vi "LUnit Configure.vi"(8 "error in (no error)":errorcluster, 9 "Default Path":path, 10 "Interactive?":bool, 11 "Coverage Report In":refnum<class "Coverage Report.lvclass">) -> (0 "error out":errorcluster, 3 "Coverage Report Out":refnum<class "Coverage Report.lvclass">)   [LabVIEW 2020, in "Coverage Report.lvclass"]
uses:
  Coverage Report.lvclass
  Coverage Report.lvclass/Coverage Report.ctl
  f97740a0-8655-44de-873d-fc598e584b33.vi
  <vilib>/Astemes/LUnit/Framework/LUnit Configuration Manager.lvclass
  <vilib>/Astemes/DevEnv/Styling/Color Theme.lvlib
panel:
  in  "VI tree":string[](tree)
  out "Coverage Include File Path":path
  in  "Report Path":path
  in  "Cancel":bool
  in  "Open New Reports":bool
  in  "Open Result in UI":bool
  in  "Commit":bool
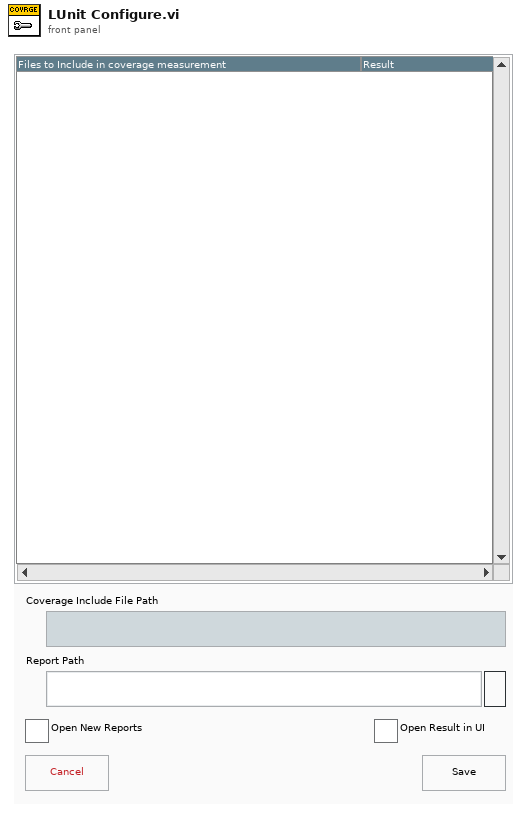
[diagram p1: front panel]
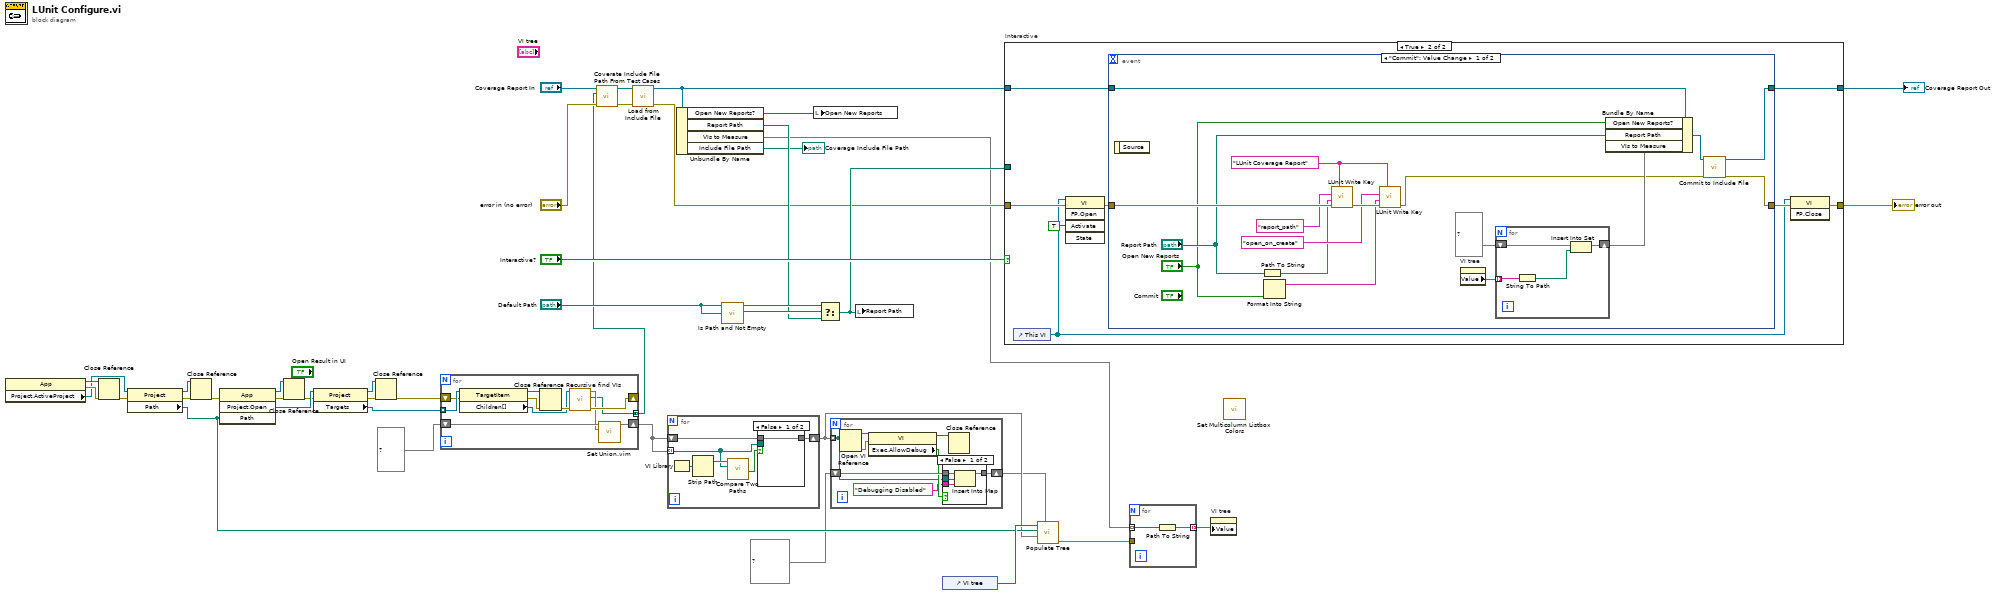
[diagram p0: block diagram]
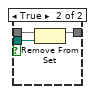
[diagram p3: hidden frame]
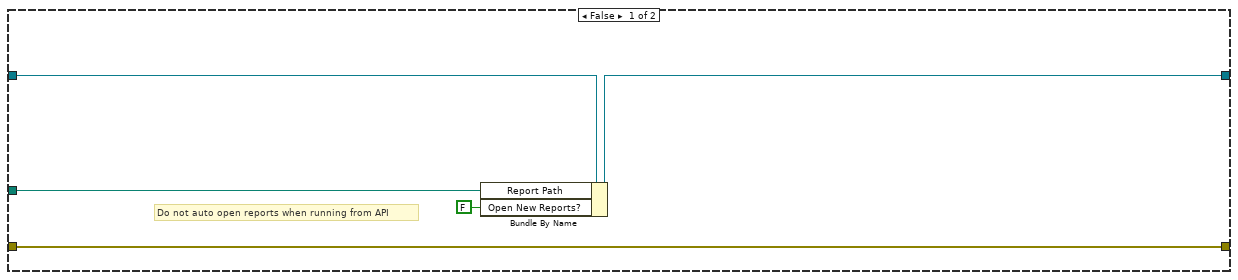
[diagram p4: hidden frame]
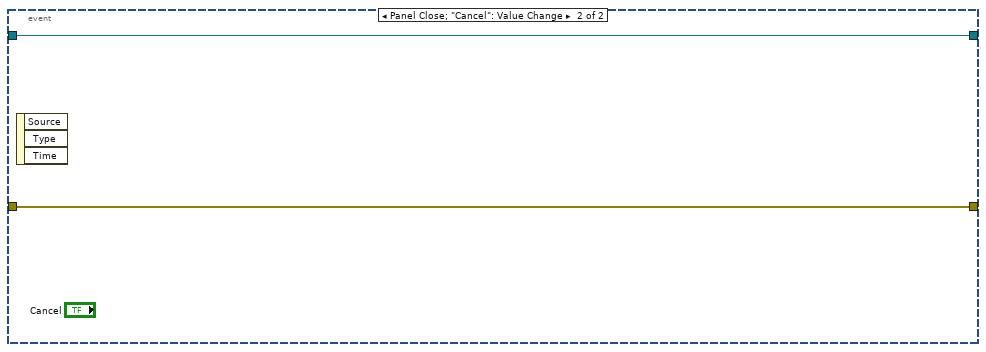
[diagram p5: hidden frame]
diagram:
  n1 = property class="App"() -> (reference out=w19:refnum<vi>, error out=w22:errorcluster, "Project.ActiveProject"=w18:refnum<vi>)  [unwired: 2 in]
  n2 = Close Reference(reference=w19, error in (no error)=w22) -> (error out=w23:errorcluster)
  n3 = property class="Project"(reference=w18, error in=w23) -> (reference out=w20:refnum<vi>, error out=w21:errorcluster, "Path"=w5:path)
  n4 = Close Reference(reference=w20, error in (no error)=w21) -> (error out=w24:errorcluster)
  n5 = invoke class="App" method="Project.Open"(error in=w24, "Path"=w5) -> (reference out=w27:refnum<vi>, error out=w31:errorcluster, "Project:Open"=w33:refnum<vi>)  [unwired: 2 in, 1 out]
  n6 = Close Reference(reference=w27, error in (no error)=w31) -> (error out=w28:errorcluster)
  n7 = property class="Project"(reference=w33, error in=w28) -> (reference out=w29:refnum<vi>, error out=w32:errorcluster, "Targets"=w25:refnum<vi>[])
  n8 = Close Reference(reference=w29, error in (no error)=w32) -> (error out=w30:errorcluster)
  n9 = for {
    tunnel: w25 -> [w52] mode=indexing
    shift-right: [w49] -> _
    shift-left: w30 -> [w50]
    shift-right: [w45] -> w8
    shift-left: set{path} {} ("VIs") -> [w47]
    tunnel: [w42] -> w11 mode=concatenating
    n10 = property class="TargetItem"(reference=w52, error in=w50) -> (reference out=w48:refnum<vi>, error out=w51:errorcluster, "Children[]"=w43:refnum<vi>[])
    n11 = Close Reference(reference=w48, error in (no error)=w51) -> (error out=w44:errorcluster)
    n12 = call "Recursive find VIs.vi"("error in (no error)"=w44, "Project Items"=w43) -> ("error out"=w49:errorcluster, "Test Case Classes"=w42:path[], "VIs"=w46:set{path})  [unwired: 7 in]
    n13 = call "Set Union.vim"("set 2"=w46, "set 1"=w47) -> ("union"=w45:set{path})  [unwired: 9 in]
  }
  n14 = call "Coverate Include File Path From Test Cases.vi"("error in (no error)"="error in (no error)", "Test Case Classes"=w11, "Coverage Report.lvclass"="Coverage Report In") -> ("error out"=w16:errorcluster, "Coverage Report.lvclass 2"=w17:refnum<class "Coverage Report.lvclass">)  [unwired: 7 in]
  n15 = call "Load from Include File.vi"("error in (no error)"=w16, "Coverage Report in"=w17) -> ("error out"=w12:errorcluster, "Coverage Report out"=w14:refnum<class "Coverage Report.lvclass">)  [unwired: 8 in]
  n16 = for {
    tunnel: w8 -> [w55] mode=indexing
    shift-right: [w54] -> w3
    shift-left: w8 -> [w56]
    n17 = VI Library() -> (path=w57:path)
    n18 = Strip Path(path=w57) -> (stripped path=w58:path)  [unwired: 1 out]
    n19 = call <vilib>:"Compare Two Paths.vi"("Path 2"=w55, "Path 1"=w58) -> ("Path 2 Relative to Path 1?"=w53:bool)  [unwired: 6 in, 3 out]
    n20 = case shown="False" w53 {
      tunnel: w56 -> [w59 w62]
      tunnel: w55 -> [_ w61]
      tunnel: [w59 w60] -> w54
      frame False {
      }
      frame True {
        n21 = Remove From Set(10:w61, 11:w62) -> (3:w60:set{path})  [unwired: 1 out]
      }
    }
  }
  n22 = Unbundle By Name(w14) -> ("Open New Reports?"=w34:bool, "Report Path"=w35:path, "VIs to Measure"=w6:set{path}, "Include File Path"=→"Coverage Include File Path":path)
  n23 = call <vilib>:"Is Path and Not Empty.vi"("path"="Default Path") -> ("Is Path and Not Empty?"=w38:bool)  [unwired: 4 in]
  n24 = local write "Open New Reports"(w34) -> ()
  n25 = Select(t="Default Path", s=w38, f=w35) -> (s? t:f=w37:path)
  n26 = for {
    tunnel: w3 -> [w64] mode=indexing
    shift-right: [w65] -> w1
    shift-left: map{path, string} {} ("Results") -> [w69]
    n27 = Open VI Reference(vi path=w64) -> (vi reference=w70:refnum<vi>, error out=w67:errorcluster)  [unwired: 5 in]
    n28 = property class="VI"(reference=w70, error in=w67) -> (reference out=w68:refnum<vi>, "Exec.AllowDebug"=w66:bool)  [unwired: 1 out]
    n29 = case shown="False" w66 {
      tunnel: w69 -> [w74 w75]
      tunnel: [w73 w75] -> w65
      tunnel: w64 -> [w72 _]
      tunnel: "Debugging Disabled" ("value") -> [w71 _]
      frame False {
        n30 = Insert Into Map(map in=w74, key=w72, value=w71) -> (map out=w73:map{path, string})  [unwired: 2 out]
      }
      frame True {
      }
    }
    n31 = Close Reference(reference=w68) -> ()  [unwired: 1 in, 1 out]
  }
  n32 = local write "Report Path"(w37) -> ()
  n33 = control-ref of="VI tree"() -> (w9:refnum<vi>)
  n34 = case "Interactive" shown="True" "Interactive?" {
    tunnel: w12 -> [w80 w86]
    tunnel: [w80 w84] -> w41
    tunnel: w14 -> [w79 w81]
    tunnel: [w78 w82] -> w39
    tunnel: w37 -> [w77 _]
    frame False {
      # "Do not auto open reports when running from API"
      n35 = Bundle By Name(cluster=w79, "Report Path"=w77, "Open New Reports?"=FALSE) -> (w78:refnum<class "Coverage Report.lvclass">)
    }
    frame True {
      n36 = control-ref of="This VI"() -> (w83:refnum<vi>)
      n37 = invoke class="VI" method="FP.Open"(reference=w83, error in=w86, "Activate"=TRUE ("Activate?")) -> (error out=w87:errorcluster)  [unwired: 2 in, 4 out]
      n38 = event shown="[0] \"Commit\": Value Change" {
        selector: _ -> [_ _]
        dyn-events: _ -> [_ _]
        timeout: _ -> [_ _]
        tunnel: w87 -> [w105 w111]
        tunnel: [w92 w111] -> w85
        tunnel: w81 -> [w99 w110]
        tunnel: [w93 w110] -> w82
        event "Commit": Value Change {
          w90 = "LUnit Coverage Report"
          n39 = event-data() -> ()  [unwired: 1 in, 1 out]
          n40 = Path To String(path="Report Path") -> (string=w101:string)
          n41 = Format Into String("Open New Reports") -> (resulting string=w100:string)  [unwired: 3 in, 1 out]
          n42 = call <vilib>:"LUnit Write Key.vi"("section"=w90, "error in (no error)"=w105, "value"=w101, "key"="report_path" ("Name")) -> ("error out"=w104:errorcluster)  [unwired: 7 in]
          n43 = call <vilib>:"LUnit Write Key.vi"("section"=w90, "error in (no error)"=w104, "value"=w100, "key"="open_on_create" ("Name")) -> ("error out"=w91:errorcluster)  [unwired: 7 in]
          n44 = property on="VI tree" class="Tree (strict)"() -> ("Value"=w89:string[])  [unwired: 2 in, 2 out]
          n45 = for {
            shift-right: [w108] -> w94
            shift-left: set{path} {} ("VIs to Measure") -> [w109]
            tunnel: w89 -> [w107] mode=indexing
            n46 = String To Path(string=w107) -> (path=w106:path)
            n47 = Insert Into Set(10:w106, 11:w109) -> (3:w108:set{path})  [unwired: 1 out]
          }
          n48 = Bundle By Name(cluster=w99, "Open New Reports?"="Open New Reports", "Report Path"="Report Path", "VIs to Measure"=w94) -> (w98:refnum<class "Coverage Report.lvclass">)
          n49 = call "Commit to Include File.vi"("error in (no error)"=w91, "Coverage Report in"=w98) -> ("error out"=w92:errorcluster, "Coverage Report out"=w93:refnum<class "Coverage Report.lvclass">)  [unwired: 8 in]
        }
        event Panel Close; "Cancel": Value Change {
          n50 = event-data() -> ()  [unwired: 1 in, 3 out]
        }
      }
      n51 = invoke class="VI" method="FP.Close"(reference=w83, error in=w85) -> (error out=w84:errorcluster)  [unwired: 1 in, 2 out]
    }
  }
  "error out" <- w41
  "Coverage Report Out" <- w39
  n52 = call "Populate Tree.vi"("Results"=w1, "VIs"=w3, "Project Path"=w5, "TreeControl in"=w9) -> ("error out"=w4:errorcluster)  [unwired: 7 in]
  n53 = for {
    tunnel: w6 -> [w113] mode=indexing
    tunnel: [w112] -> w7 mode=indexing
    tunnel: w4 -> [_]
    n54 = Path To String(path=w113) -> (string=w112:string)
  }
  n55 = property on="VI tree" class="Tree (strict)"("Value"=w7) -> ()  [unwired: 2 in, 2 out]
  n56 = call <vilib>:"Set Multicolumn Listbox Colors.vi"() -> ()  [unwired: 11 in, 1 out]
